vi "NextUpSgl.vi"(11 "Value":sgl format="%#_13g") -> (3 "NextUp":sgl format="%#_29e")   [LabVIEW 2019, in "FloatUtil.lvlib"]
uses:
  FloatUtil.lvlib
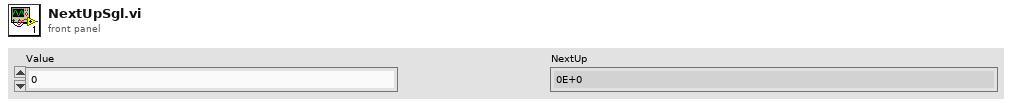
[diagram p1: front panel]
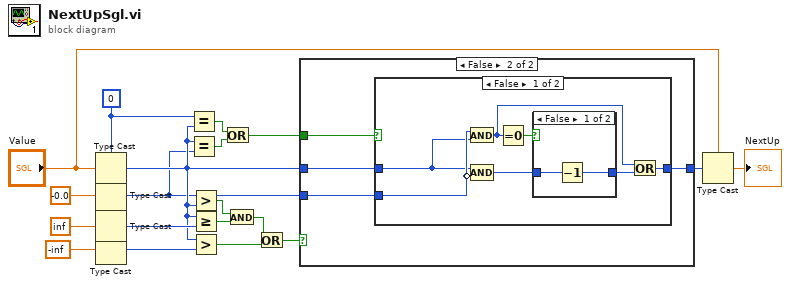
[diagram p0: block diagram]
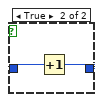
[diagram p3: hidden frame]
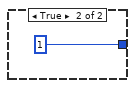
[diagram p4: hidden frame]
diagram:
  w6 = u32 0
  n1 = Type Cast(type=w6, x="Value") -> (*(type *) &x=w5:u32)
  n2 = Type Cast(type=w6, x=sgl -0.0 ("Value")) -> (*(type *) &x=w4:u32)
  n3 = Type Cast(type=w6, x=sgl inf ("Value")) -> (*(type *) &x=w8:u32)
  n4 = Type Cast(type=w6, x=sgl -inf ("Value")) -> (*(type *) &x=w7:u32)
  n5 = Equal?(x=w6, y=w5) -> (x = y?=w2:bool)
  n6 = Equal?(x=w5, y=w4) -> (x = y?=w3:bool)
  n7 = Greater?(x=w4, y=w5) -> (0:w18:bool)
  n8 = Greater Or Equal?(x=w5, y=w8) -> (x >= y?=w19:bool)
  n9 = Greater?(x=w5, y=w7) -> (0:w16:bool)
  n10 = Or(x=w2, y=w3) -> (x .or. y?=w1:bool)
  n11 = And(x=w18, y=w19) -> (x .and. y?=w17:bool)
  n12 = Or(x=w17, y=w16) -> (x .or. y?=w15:bool)
  n13 = case shown="False" w15 {
    tunnel: w5 -> [w20 w21]
    tunnel: [w20 w24] -> w14
    tunnel: w4 -> [_ w23]
    tunnel: w1 -> [_ w22]
    frame True {
    }
    frame False {
      n14 = case shown="False" w22 {
        tunnel: [w28 u32 1] -> w24
        tunnel: w23 -> [w26 _]
        tunnel: w21 -> [w25 _]
        frame False {
          n15 = And(x=w26, y=w25) -> (x .and. y?=w27:u32)
          n16 = Compound Arithmetic op=AND(w25, invert w26) -> (w30:u32)
          n17 = Equal To 0?(x=w27) -> (x = 0?=w31:bool)
          n18 = case shown="False" w31 {
            tunnel: w30 -> [w33 w35]
            tunnel: [w32 w34] -> w29
            frame False {
              n19 = Decrement(x=w33) -> (x-1=w32:u32)
            }
            frame True {
              n20 = Increment(x=w35) -> (x+1=w34:u32)
            }
          }
          n21 = Or(x=w27, y=w29) -> (x .or. y?=w28:u32)
        }
        frame True {
        }
      }
    }
  }
  n22 = Type Cast(type="Value", x=w14) -> (*(type *) &x=→"NextUp":sgl)
